vi "20151104 pulse limiter.vi"(4 "Pulse in":u16) -> (2 "Pulse out":u16)   [LabVIEW 2013]
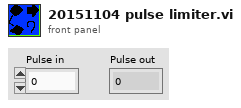
[diagram p1: front panel]
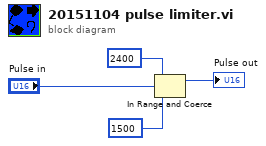
[diagram p0: block diagram]
diagram:
  n1 = In Range and Coerce(upper limit=u16 2400, x="Pulse in", lower limit=u16 1500) -> (coerced(x)=→"Pulse out":u16)  [unwired: 1 out]
